vi "feladat_3).vi"() -> (1 "number":i64, 2 "Array":i64[](array[numeric]), 3 "Boolean":bool)   [LabVIEW 2021]
uses:
  <vilib>/numeric/Random Number (Range) I64.vi
  <vilib>/numeric/sub_Random U32.vi
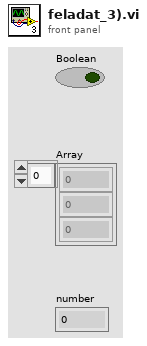
[diagram p1: front panel]
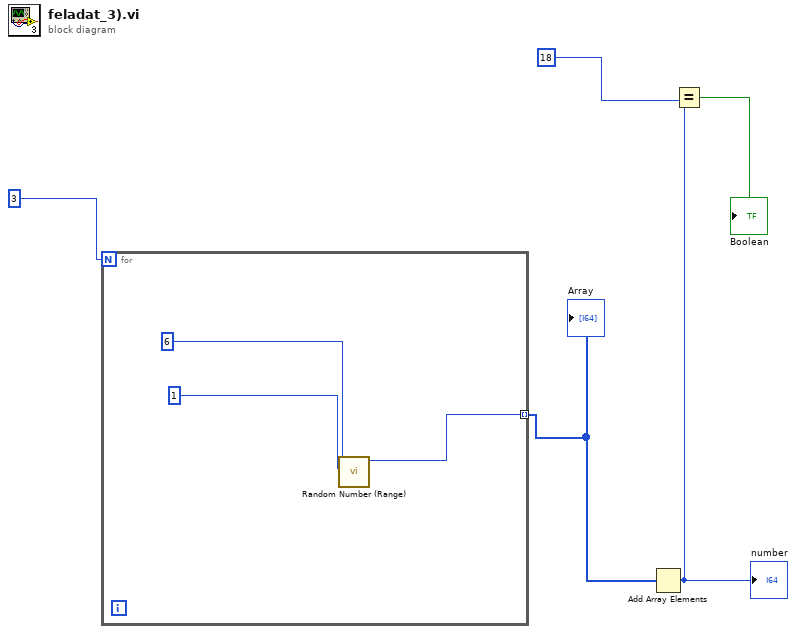
[diagram p0: block diagram]
diagram:
  n1 = for {
    N: 3 -> [_]
    tunnel: [w6] -> w2 mode=indexing
    n2 = call-poly <vilib>:"Random Number (Range).vi"("lower bound (-100)"=1, "upper bound (100)"=6) -> ("number"=w6:i64)  [unwired: 9 in]
  }
  "Array" <- w2
  n3 = Add Array Elements(numeric array=w2) -> (sum=w3:i64)
  "number" <- w3
  n4 = Equal?(x=w3, y=18) -> (x = y?=→"Boolean":bool)
